vi "4ndOrderDerivate.vi"(8 "error in (no error)":errorcluster, 9 "dt":dbl=1.0 format="%0.2f", 10 "x":dbl format="%0.2f", 11 "Utilities in":refnum<class "Utilities.lvclass">) -> (0 "error out":errorcluster, 2 "dx/dt":dbl format="%0.2f", 3 "Utilities out":refnum<class "Utilities.lvclass">)   [LabVIEW 2018, in "Utilities.lvclass"]
uses:
  Utilities.lvclass
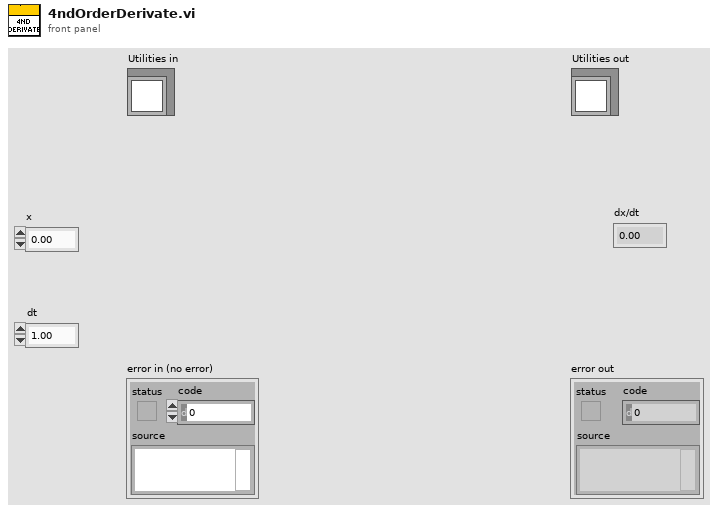
[diagram p1: front panel]
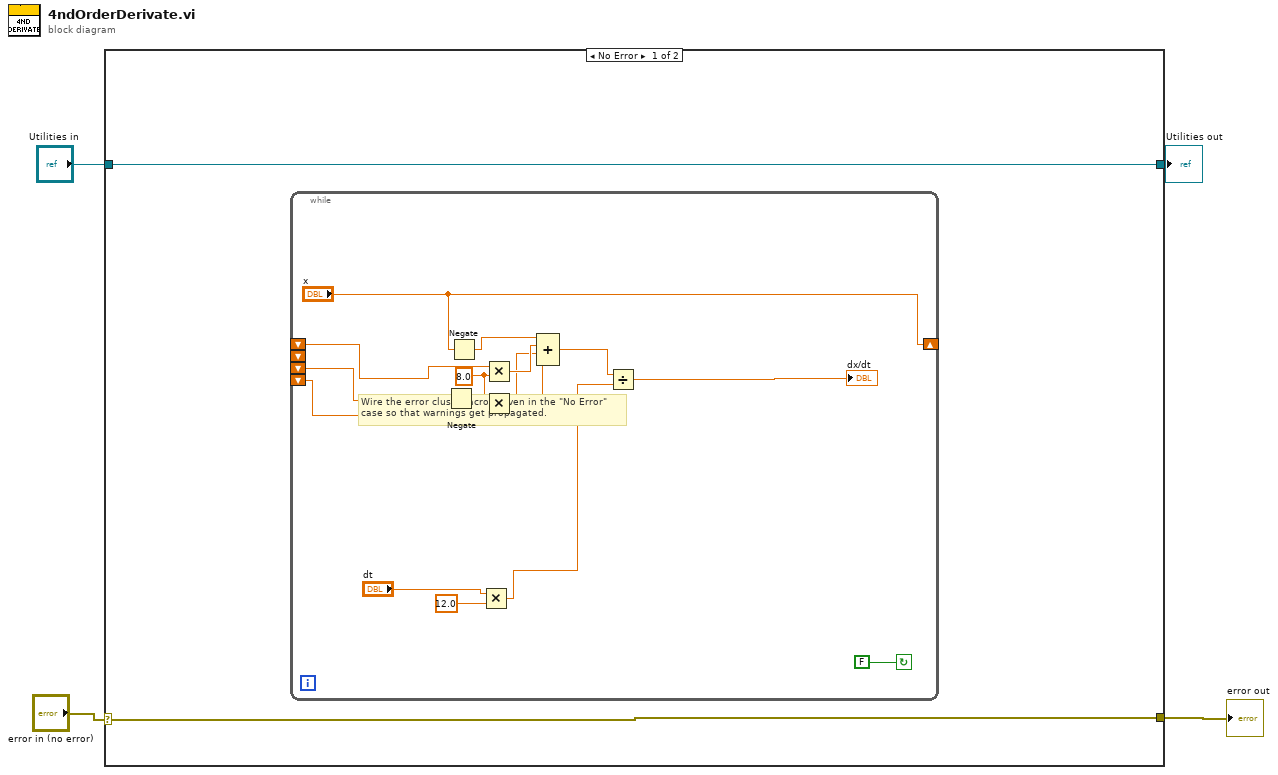
[diagram p0: block diagram]
diagram:
  n1 = case shown="No Error" "error in (no error)" {
    selector: "error in (no error)" -> [w5 w23]
    tunnel: [w5 w23] -> w3
    tunnel: [w6 w22] -> w1
    tunnel: "Utilities in" -> [w6 w22]
    frame No Error {
      # "Wire the error cluster across even in the \"No Error\"\ncase so that warnings get propagated."
      n2 = while {
        shift-left: _ -> [_]
        shift-left: _ -> [w18]
        shift-right: ["x"] -> _
        shift-left: _ -> [w15]
        shift-left: _ -> [w16]
        stop <- FALSE continue-if-true
        w11 = 8.0 ("y")
        n3 = Negate(x=w15) -> (-x=w12:dbl)
        n4 = Negate(x="x") -> (-x=w10:dbl)
        n5 = Multiply(x="dt", y=12.0) -> (x*y=w13:dbl)
        n6 = Multiply(x=w18, y=w11) -> (x*y=w9:dbl)
        n7 = Multiply(x=w12, y=w11) -> (x*y=w8:dbl)
        n8 = Compound Arithmetic op=ADD(w10, w9, w8, w16) -> (w7:dbl)
        n9 = Divide(x=w7, y=w13) -> (x/y=→"dx/dt":dbl)
      }
    }
    frame Error {
    }
  }
  "error out" <- w3
  "Utilities out" <- w1
